vi "login.vi"() -> ()   [LabVIEW 2014]
panel:
  in  "布尔":bool
  in  "密码":string="password"
  in  "用户名":string="username"
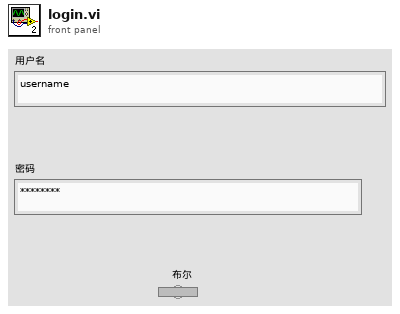
[diagram p1: front panel]
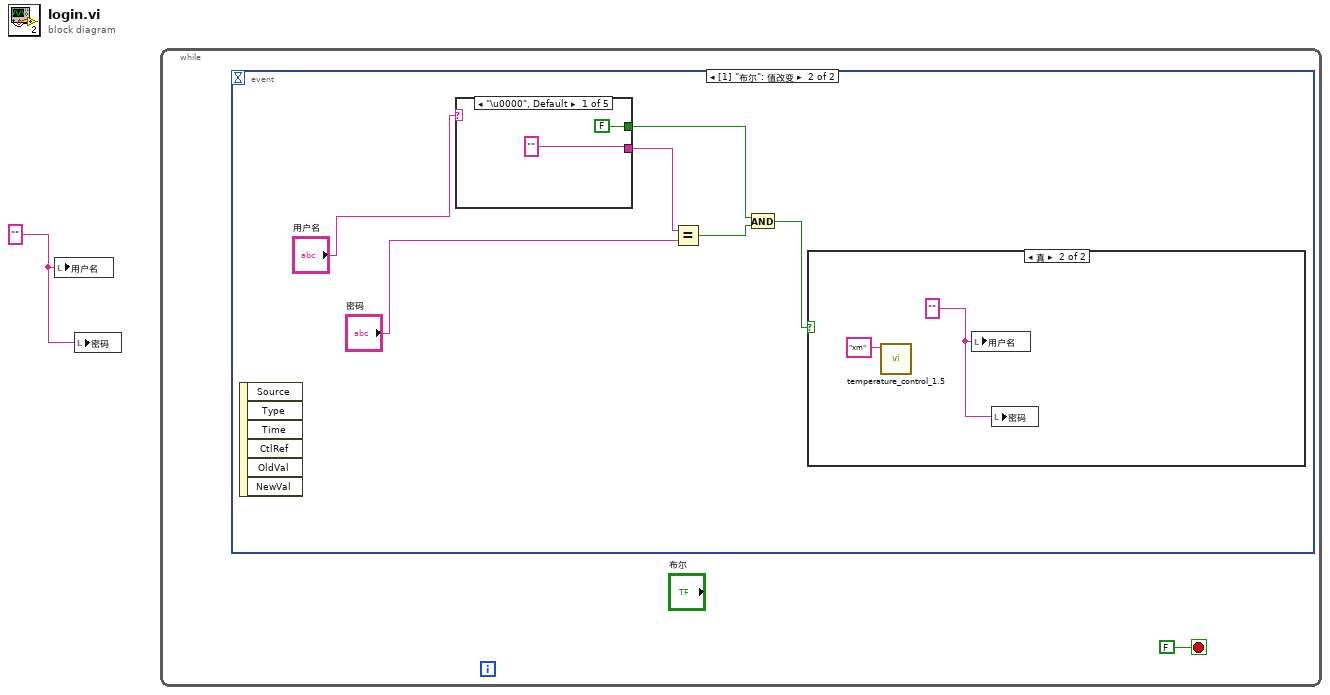
[diagram p0: block diagram]
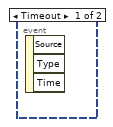
[diagram p2: hidden frame]
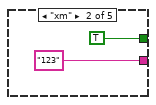
[diagram p3: hidden frame]
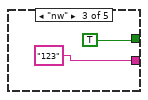
[diagram p4: hidden frame]
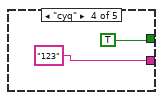
[diagram p5: hidden frame]
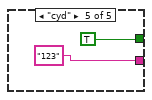
[diagram p6: hidden frame]
diagram:
  w1 = ""
  n1 = local write "用户名"(w1) -> ()
  n2 = local write "密码"(w1) -> ()
  n3 = while {
    stop <- FALSE stop-if-true
    n4 = event shown="[1] \"布尔\": 值改变" {
      selector: _ -> [_ _]
      dyn-events: _ -> [_ _]
      timeout: _ -> [_ _]
      event Timeout {
        n5 = event-data() -> ()  [unwired: 1 in, 3 out]
      }
      event "布尔": Value Change {
        n6 = event-data() -> ()  [unwired: 1 in, 6 out]
        n7 = case shown="\"\", 默认" "用户名" {
          tunnel: ["" "123" "123" "123" "123"] -> w6
          tunnel: [FALSE TRUE TRUE TRUE TRUE] -> w4
          frame "\u0000", Default {
          }
          frame "xm" {
          }
          frame "nw" {
          }
          frame "cyq" {
          }
          frame "cyd" {
          }
        }
        n8 = Equal?(x=w6, y="密码") -> (x = y?=w5:bool)
        n9 = And(x=w4, y=w5) -> (x .and. y?=w3:bool)
        n10 = case shown="真" w3 {
          frame False {
          }
          frame True {
            w20 = ""
            n11 = call "temperature_control_1.5.vi"("User"="xm") -> ()  [unwired: 11 in]
            n12 = local write "用户名"(w20) -> ()
            n13 = local write "密码"(w20) -> ()
          }
        }
      }
    }
  }
